vi "TL_read_laser_cluster.vi"(6 "Global parameters":T1={"405"=0.0, "488"=0.0, "561"=0.0, "641"=0.0, "BF"=0.0, "X"=0.0, "Y"=0.0, "Filter list"=1, "Exp time"=0.0, "Kinetic time"=0.0, "Gain"=0, "Step length (nm)"=0, "Total range (nm)"=0, "Scan illumination\n mode"=FALSE, "Dt (s)"=0, "# repetitions"=0} {"# repetitions" min=0; "Dt (s)" min=0 step=1; "Filter list" items=["ET665lp", "zet405/488/561/640m", "None", "None", "None", "None"]}, 7 "TL movie path":path, 8 "error in":errorcluster caption="error in (no error)", 10 "TL - Laser cluster":T2={"405"=0.0, "488"=0.0, "561"=0.0, "641"=0.0, "BF "=0.0, "405 setpoint"=FALSE, "488 setpoint"=FALSE, "561 setpoint"=FALSE, "641 setpoint"=FALSE, "BF setpoint"=FALSE, "N planes 405"=0, "Dz 405"=0, "N planes 488"=0, "Dz 488"=0, "N planes 561"=0, "Dz 561"=0, "N planes 641"=0, "Dz 641"=0, "N planes BF"=0, "Dz BF"=0, "Tau 405"=inf, "Tau 488"=inf, "Tau 561"=inf, "Tau 641"=inf, "Tau BF"=inf, "405 set"=FALSE, "488 set "=FALSE, "561 set"=FALSE, "641 set"=FALSE, "BF set"=FALSE} {"Tau BF" format="%#_6e"; "Tau 641" format="%#_6e"; "Tau 561" format="%#_6e"; "Tau 488" format="%#_6e"; "Tau 405" format="%#_6e"; "641" min=0.0 max=100.0 step=0.1 scale=0.0..100.0; "561" min=0.0 max=100.0 step=0.1 scale=0.0..100.0; "405" min=0.0 max=100.0 step=0.1 scale=0.0..100.0; "488" min=0.0 max=100.0 step=0.1 scale=0.0..100.0; "BF" min=0.0 max=100.0 step=0.1 scale=0.0..100.0}, 11 "TL - setpoint cluster":T3) -> (0 "error out":errorcluster, 2 "Channel #":i32, 3 "Array":dbl[][](array[numeric]), 5 "Not empty":bool)   [LabVIEW 2015]
uses:
  CONTROLS/Time_lapse_parameters.ctl
  CONTROLS/Global parameters.ctl
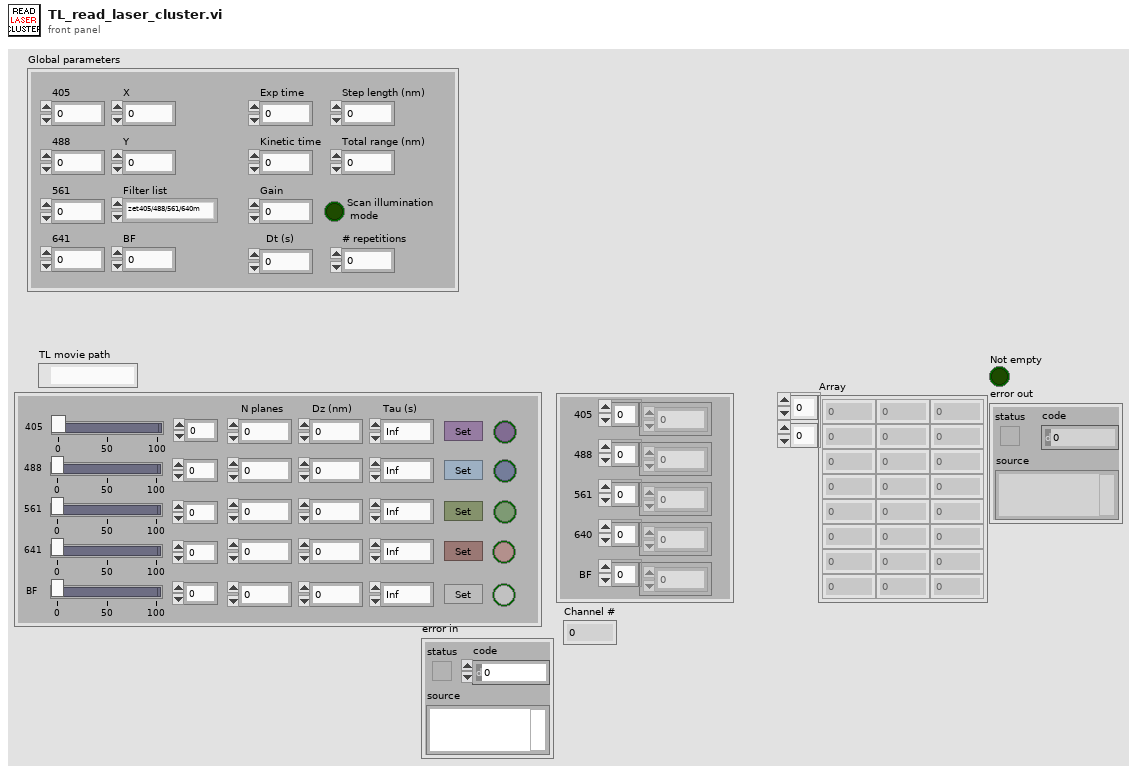
[diagram p1: front panel]
types:
  T1 = typedef "Global parameters.ctl" = cluster{"405":dbl, "488":dbl, "561":dbl, "641":dbl, "BF":dbl, "X":dbl, "Y":dbl, "Filter list":u16, "Exp time":sgl, "Kinetic time":sgl, "Gain":i32, "Step length (nm)":u32, "Total range (nm)":u32, "Scan illumination\n mode":bool, "Dt (s)":i32, "# repetitions":i32}
  T2 = typedef "Time_lapse_parameters.ctl" = cluster{"405":dbl, "488":dbl, "561":dbl, "641":dbl, "BF ":dbl, "405 setpoint":bool, "488 setpoint":bool, "561 setpoint":bool, "641 setpoint":bool, "BF setpoint":bool, "N planes 405":i32, "Dz 405":i32, "N planes 488":i32, "Dz 488":i32, "N planes 561":i32, "Dz 561":i32, "N planes 641":i32, "Dz 641":i32, "N planes BF":i32, "Dz BF":i32, "Tau 405":dbl, "Tau 488":dbl, "Tau 561":dbl, "Tau 641":dbl, "Tau BF":dbl, "405 set":bool, "488 set ":bool, "561 set":bool, "641 set":bool, "BF set":bool}
  T3 = cluster{"405":dbl[], "488":dbl[], "561":dbl[], "640":dbl[], "BF":dbl[]}
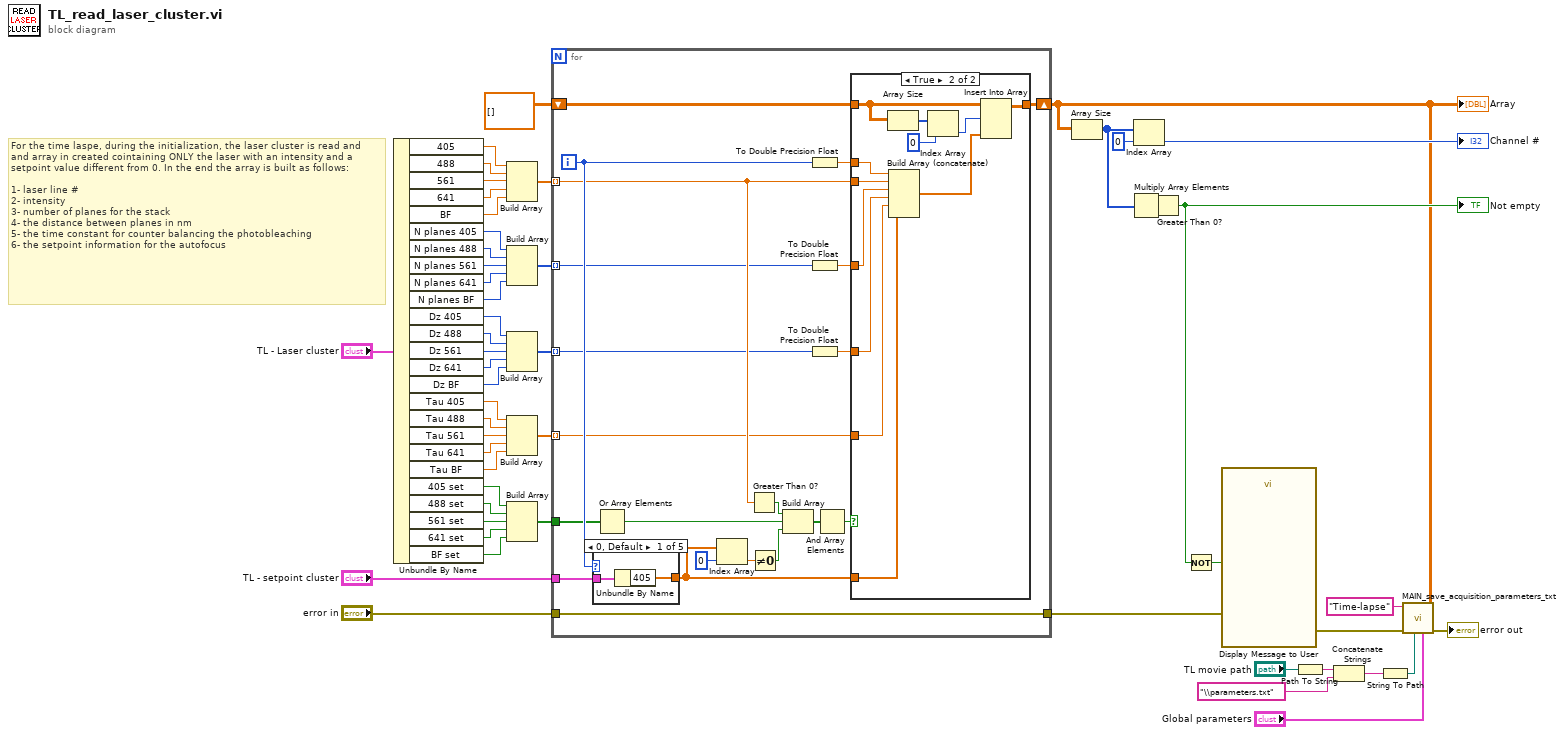
[diagram p0: block diagram]
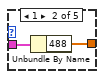
[diagram p2: hidden frame]
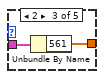
[diagram p3: hidden frame]
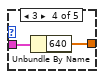
[diagram p4: hidden frame]
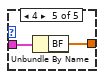
[diagram p5: hidden frame]
diagram:
  # "For the time laspe, during the initialization, the laser cluster is read and \nand array in created cointaining ONLY the laser with an intensity and a \nsetpoint value different from 0. In the end the array is built as follows:\n\n1- laser line #\n2- intensity\n3- number of planes for the stack\n4- the distance between planes in nm\n5- the time constant for counter balancing the photobleaching\n6- the setpoint information for the autofocus"
  n1 = Unbundle By Name("TL - Laser cluster") -> ("405"=w43:dbl, "488"=w42:dbl, "561"=w41:dbl, "641"=w40:dbl, "BF"=w39:dbl, "N planes 405"=w38:i32, "N planes 488"=w36:i32, "N planes 561"=w37:i32, "N planes 641"=w35:i32, "N planes BF"=w34:i32, "Dz 405"=w28:i32, "Dz 488"=w31:i32, "Dz 561"=w32:i32, "Dz 641"=w30:i32, "Dz BF"=w29:i32, "Tau 405"=w18:dbl, "Tau 488"=w19:dbl, "Tau 561"=w20:dbl, "Tau 641"=w21:dbl, "Tau BF"=w22:dbl, "405 set"=w16:bool, "488 set"=w15:bool, "561 set"=w14:bool, "641 set"=w13:bool, "BF set"=w12:bool)
  n2 = Build Array(w43, w42, w41, w40, w39) -> (w50:dbl[])
  n3 = Build Array(w38, w36, w37, w35, w34) -> (w33:i32[])
  n4 = Build Array(w28, w31, w32, w30, w29) -> (w27:i32[])
  n5 = Build Array(w18, w19, w20, w21, w22) -> (w17:dbl[])
  n6 = Build Array(w16, w15, w14, w13, w12) -> (w11:bool[])
  n7 = for {
    tunnel: w50 -> [w63] mode=indexing
    shift-right: [w71] -> w9
    shift-left: dbl[][] [] ("Array") -> [w72]
    tunnel: "TL - setpoint cluster" -> [w68]
    tunnel: "error in" -> [w70]
    tunnel: [w70] -> w45
    tunnel: w33 -> [w62] mode=indexing
    tunnel: w27 -> [w60] mode=indexing
    tunnel: w17 -> [w58] mode=indexing
    tunnel: w11 -> [w57]
    i -> [w67]
    n8 = case shown="0, Default" w67 {
      tunnel: w68 -> [w74 w76 w78 w80 w82]
      tunnel: [w73 w75 w77 w79 w81] -> w64
      frame 0, Default {
        n9 = Unbundle By Name(w74) -> ("405"=w73:dbl[])
      }
      frame 1 {
        n10 = Unbundle By Name(w76) -> ("488"=w75:dbl[])
      }
      frame 2 {
        n11 = Unbundle By Name(w78) -> ("561"=w77:dbl[])
      }
      frame 3 {
        n12 = Unbundle By Name(w80) -> ("640"=w79:dbl[])
      }
      frame 4 {
        n13 = Unbundle By Name(w82) -> ("BF"=w81:dbl[])
      }
    }
    n14 = Or Array Elements(Boolean array=w57) -> (logical OR=w55:bool)
    n15 = Index Array(array=w64, index=0) -> (element=w65:dbl)
    n16 = Greater Than 0?(x=w63) -> (x > 0?=w56:bool)
    n17 = Not Equal To 0?(x=w65) -> (x != 0?=w54:bool)
    n18 = Build Array(w56, w55, w54) -> (w53:bool[])
    n19 = To Double Precision Float(number=w67) -> (double precision float=w69:dbl)
    n20 = To Double Precision Float(number=w62) -> (double precision float=w61:dbl)
    n21 = To Double Precision Float(number=w60) -> (double precision float=w59:dbl)
    n22 = And Array Elements(Boolean array=w53) -> (logical AND=w52:bool)
    n23 = case shown="True" w52 {
      tunnel: w69 -> [_ w95]
      tunnel: w72 -> [w83 w92]
      tunnel: [w83 w93] -> w71
      tunnel: w64 -> [_ w84]
      tunnel: w63 -> [_ w88]
      tunnel: w61 -> [_ w87]
      tunnel: w59 -> [_ w86]
      tunnel: w58 -> [_ w85]
      frame False {
      }
      frame True {
        n24 = Array Size(array=w92) -> (size(s)=w91:i32[])
        n25 = Build Array (concatenate)(w95, w88, w87, w86, w85, w84) -> (w94:dbl[])
        n26 = Index Array(array=w91, index=0) -> (element=w89:i32)
        n27 = Insert Into Array(array=w92, index (row)=w89, new element=w94) -> (w93:dbl[][])  [unwired: 1 in]
      }
    }
  }
  "Array" <- w9
  n28 = Array Size(array=w9) -> (size(s)=w26:i32[])
  n29 = Multiply Array Elements(1:w26) -> (0:w49:i32)
  n30 = Index Array(array=w26, index=0) -> (element=→"Channel #":i32)
  n31 = Greater Than 0?(x=w49) -> (x > 0?=w48:bool)
  "Not empty" <- w48
  n32 = Not(x=w48) -> (.not. x?=w47:bool)
  n33 = call "Display Message to User"("error in (no error)"=w45, "Enable"=w47) -> ("error out"=w10:errorcluster)  [unwired: 8 in, 1 out]
  n34 = Path To String(path="TL movie path") -> (string=w4:string)
  n35 = Concatenate Strings(w4, "\\parameters.txt" ("string")) -> (w2:string)
  n36 = String To Path(string=w2) -> (path=w1:path)
  n37 = call "MAIN_save_acquisition_parameters_txt.vi"("TL Array"=w9, "Global parameters"="Global parameters", "file path"=w1, "error in"=w10, "Data type"="Time-lapse") -> ("error out"=→"error out":errorcluster)  [unwired: 6 in]
